vi "RW_MFG_Pack_Config.vi"(0 "configuration file path":path, 5 "Path in":path, 7 "Default in":string, 9 "Mode":enum16{"Read", "Write"}(ring), 11 "error in (no error)":errorcluster) -> (6 "Path":path, 8 "Default":string, 15 "error out":errorcluster)   [LabVIEW 2022 SP3, in "MES_Local.lvlib" / "MES_Local.lvclass"]
uses:
  MES_Local.lvclass
  <vilib>/Utility/config.llb/Read Key (Path).vi
  <vilib>/Utility/config.llb/Read Key (String).vi
  <vilib>/Utility/config.llb/Write Key (Path).vi
  <vilib>/Utility/config.llb/Write Key (String).vi
  <vilib>/Utility/config.llb/NI_LVConfig.lvlib
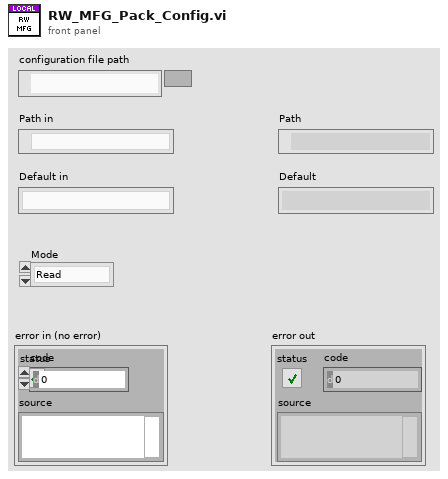
[diagram p1: front panel]
types:
  T1 = typedef "NI_LVConfig.lvlib/Config Data RefNum.ctl" = refnum<k1>
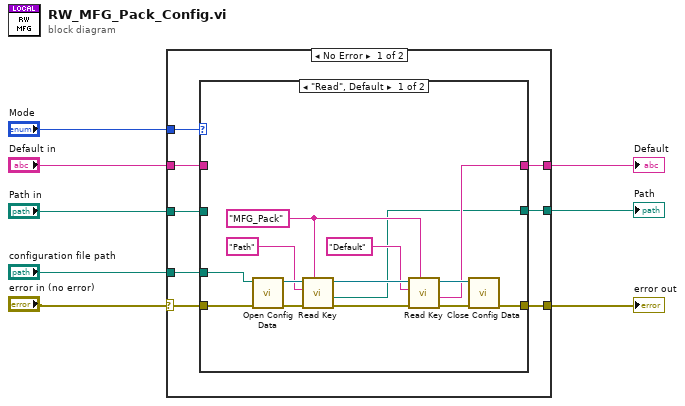
[diagram p0: block diagram]
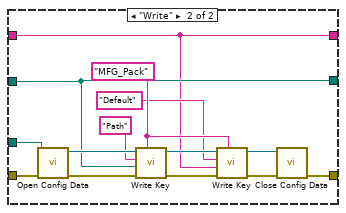
[diagram p2: hidden frame]
diagram:
  n1 = case shown="No Error" "error in (no error)" {
    selector: "error in (no error)" -> [w13 w45]
    tunnel: "configuration file path" -> [w16 _]
    tunnel: [w15 w46] -> w7
    tunnel: [w14 w45] -> w6
    tunnel: [w12 w47] -> w4
    tunnel: "Mode" -> [w11 _]
    tunnel: "Default in" -> [w10 w46]
    tunnel: "Path in" -> [w9 w47]
    frame No Error {
      n2 = case shown="\"Read\", Default" w11 {
        tunnel: w16 -> [w28 w42]
        tunnel: [w20 w31] -> w15
        tunnel: w13 -> [w19 w44]
        tunnel: [w18 w43] -> w14
        tunnel: [w17 w32] -> w12
        tunnel: w10 -> [_ w31]
        tunnel: w9 -> [_ w32]
        frame "Read", Default {
          w22 = "MFG_Pack" ("section")
          n3 = call <vilib>:"Open Config Data.vi"("error in (no error)"=w19, "configuration file path"=w28) -> ("error out"=w30:errorcluster, "refnum"=w29:T1)  [unwired: 7 in, 1 out]
          n4 = call-poly <vilib>:"Read Key.vi"("section"=w22, "error in (no error)"=w30, "key"="Path", "refnum"=w29) -> ("error out"=w26:errorcluster, "value"=w17:path, "refnum out"=w25:T1)  [unwired: 4 in, 1 out]
          n5 = call-poly <vilib>:"Read Key.vi"("section"=w22, "error in (no error)"=w26, "key"="Default", "refnum"=w25) -> ("error out"=w24:errorcluster, "value"=w20:string, "refnum out"=w23:T1)  [unwired: 4 in, 1 out]
          n6 = call <vilib>:"Close Config Data.vi"("error in (no error)"=w24, "refnum"=w23) -> ("error out"=w18:errorcluster)  [unwired: 8 in, 1 out]
        }
        frame "Write" {
          w35 = "MFG_Pack" ("section")
          n7 = call <vilib>:"Open Config Data.vi"("error in (no error)"=w44, "configuration file path"=w42) -> ("error out"=w40:errorcluster, "refnum"=w38:T1)  [unwired: 7 in, 1 out]
          n8 = call-poly <vilib>:"Write Key.vi"("section"=w35, "error in (no error)"=w40, "value"=w32, "key"="Path", "refnum"=w38) -> ("error out"=w41:errorcluster, "refnum out"=w37:T1)  [unwired: 4 in, 1 out]
          n9 = call-poly <vilib>:"Write Key.vi"("section"=w35, "error in (no error)"=w41, "value"=w31, "key"="Default", "refnum"=w37) -> ("error out"=w39:errorcluster, "refnum out"=w36:T1)  [unwired: 4 in, 1 out]
          n10 = call <vilib>:"Close Config Data.vi"("error in (no error)"=w39, "refnum"=w36) -> ("error out"=w43:errorcluster)  [unwired: 8 in, 1 out]
        }
      }
    }
    frame Error {
    }
  }
  "Default" <- w7
  "Path" <- w4
  "error out" <- w6
